vi "flattenPressureToXML_Scalar.vi"(8 "error in (no error)":errorcluster, 9 "pressureUnitInXML":T1, 10 "pressureAgain":variant, 11 "pressure":dbl[unit]) -> (0 "error out":errorcluster, 3 "xmlString":string)   [LabVIEW 2016, in "UnitsAndXML.lvlib"]
uses:
  <userlib>/Common/UnitsAndXML/UnitsAndXML.lvlib
  <userlib>/Common/UnitsAndXML/FlattenItemWithUnitToXML/FlattenPressureToXML/PressureUnit.ctl
  <vilib>/Utility/VariantDataType/VariantType.lvlib
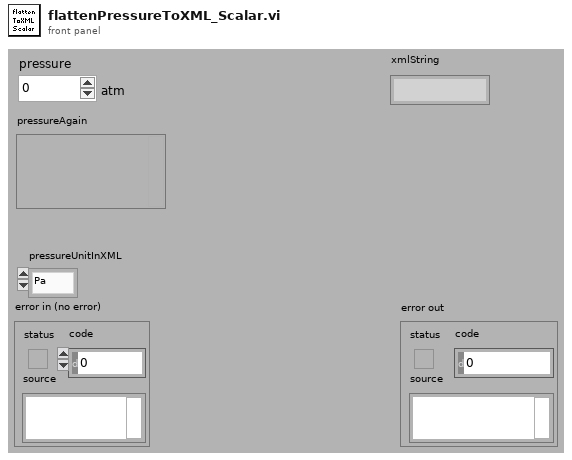
[diagram p1: front panel]
types:
  T1 = typedef "UnitsAndXML.lvlib/PressureUnit.ctl" = enum16{"Pa", "atm", "bar", "mbar", "m.Hg", "psi", "torr"}
  T2 = typedef "VariantType.lvlib/Type.ctl" = enum8{"Invalid Type", "Void", "I8", "I16", "I32", "I64", "U8", "U16", "U32", "U64", "Single Float", "Double Float", "Extended Float", "Single Complex", "Double Complex", "Extended Complex", "Enum U8", "Enum U16", "Enum U32", "Enum U64", "Single Float With Unit", "Double Float With Unit", "Extended Float With Unit", "Single Complex with Unit", "Double Complex with Unit", "Extended Complex with Unit", "Boolean", "String", "Path", "Picture", "Tag", "Array", "Cluster", "Variant", "LV Variant", "Waveform", "Timestamp", "Digital Waveform", "Digital Data", "ExpressData", "Refnum", "External Data", "VI", "Poly VI", "LabVIEW Class Instance", "Fixed Point"}
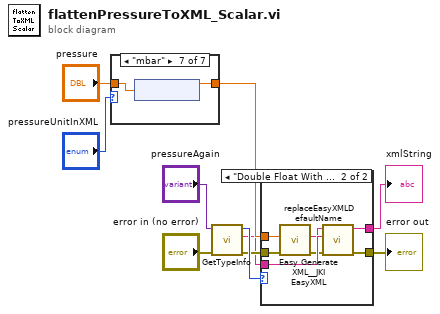
[diagram p0: block diagram]
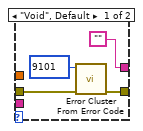
[diagram p2: hidden frame]
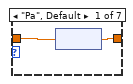
[diagram p3: hidden frame]
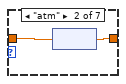
[diagram p4: hidden frame]
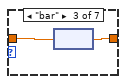
[diagram p5: hidden frame]
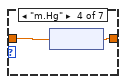
[diagram p6: hidden frame]
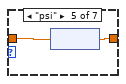
[diagram p7: hidden frame]
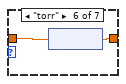
[diagram p8: hidden frame]
diagram:
  n1 = case shown="\"mbar\"" "pressureUnitInXML" {
    tunnel: "pressure" -> [w12 w14 w16 w18 w20 w22 w24]
    tunnel: [w11 w13 w15 w17 w19 w21 w23] -> w10
    frame "Pa", Default {
      n2 = node(w12) -> (w11:dbl)
    }
    frame "atm" {
      n3 = node(w14) -> (w13:dbl)
    }
    frame "bar" {
      n4 = node(w16) -> (w15:dbl)
    }
    frame "m.Hg" {
      n5 = node(w18) -> (w17:dbl)
    }
    frame "psi" {
      n6 = node(w20) -> (w19:dbl)
    }
    frame "torr" {
      n7 = node(w22) -> (w21:dbl)
    }
    frame "mbar" {
      n8 = node(w24) -> (w23:dbl)
    }
  }
  n9 = call <vilib>:"GetTypeInfo.vi"("error in (no error)"="error in (no error)", "Variant"="pressureAgain") -> ("error out"=w2:errorcluster, "Name"=w1:string, "Type Enum"=w3:T2)  [unwired: 5 in, 2 out]
  n10 = case shown="\"Double Float With Unit\"" w3 {
    tunnel: w10 -> [_ w35]
    tunnel: ["" w34] -> w7
    tunnel: [w27 w33] -> w6
    tunnel: w2 -> [w25 w30]
    tunnel: w1 -> [_ w32]
    frame "Void", Default {
      n11 = call <vilib>:"Error Cluster From Error Code.vi"("error in (no error)"=w25, "error code (0)"=9101) -> ("error out"=w27:errorcluster)  [unwired: 7 in]
    }
    frame "Double Float With Unit" {
      n12 = call <vilib>:"Easy Generate XML__JKI EasyXML.vi"("error in (no error)"=w30, "LabVIEW Data"=w35) -> ("error out"=w29:errorcluster, "XML String"=w31:string)  [unwired: 8 in]
      n13 = call <userlib>:"replaceEasyXMLDefaultName.vi"("error in"=w29, "desiredName"=w32, "easyXMLStringWithDefaultNames"=w31) -> ("error out"=w33:errorcluster, "xmlString"=w34:string)  [unwired: 7 in]
    }
  }
  "xmlString" <- w7
  "error out" <- w6
